vi "Level Function with Limits.vi"() -> ()   [LabVIEW 2014]
panel:
  in  "Bottom":bool
  in  "Top":bool
  out "Motor Value":dbl
  out "Is Below":bool
  out "Is Above":bool
  in  "stop":bool
  out "coerced(x)":dbl
  out "In Range?":bool
  in  "Input":dbl(slide) scale=0.0..20.0
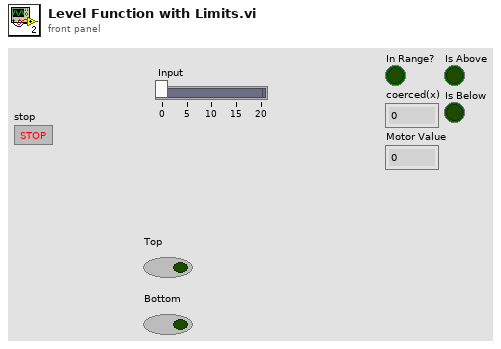
[diagram p1: front panel]
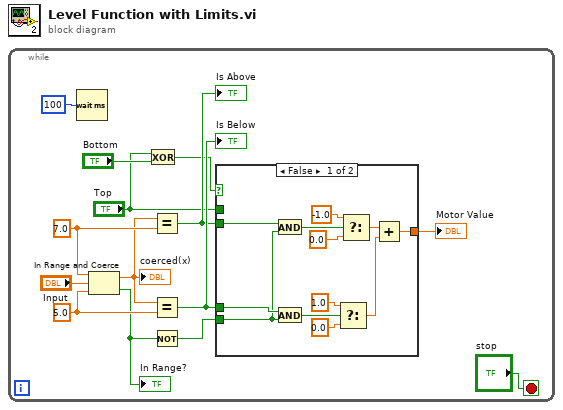
[diagram p0: block diagram]
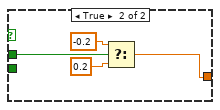
[diagram p2: hidden frame]
diagram:
  n1 = while {
    stop <- "stop" stop-if-true
    w10 = 5.0 ("upper limit")
    w11 = 7.0 ("upper limit")
    n2 = Wait (ms)(milliseconds to wait=u32 100) -> ()  [unwired: 1 out]
    n3 = In Range and Coerce(upper limit=w11, x="Input", lower limit=w10) -> (coerced(x)=w9:dbl, In Range?=w6:bool)
    "In Range?" <- w6
    "coerced(x)" <- w9
    n4 = Exclusive Or(1:"Bottom", 2:"Top") -> (0:w2:bool)
    n5 = Equal?(x=w9, y=w11) -> (x = y?=w7:bool)
    "Is Above" <- w7
    n6 = Equal?(x=w9, y=w10) -> (x = y?=w8:bool)
    "Is Below" <- w8
    n7 = Not(x=w6) -> (.not. x?=w5:bool)
    n8 = case shown="False" w2 {
      tunnel: w8 -> [w17 _]
      tunnel: w7 -> [w18 _]
      tunnel: w5 -> [w16 _]
      tunnel: [w15 w30] -> w4
      tunnel: "Top" -> [_ w29]
      frame False {
        n9 = And(x=w18, y=w16) -> (x .and. y?=w26:bool)
        n10 = And(x=w17, y=w16) -> (x .and. y?=w25:bool)
        n11 = Select(t=1.0, s=w25, f=0.0) -> (s? t:f=w19:dbl)
        n12 = Select(t=-1.0, s=w26, f=0.0) -> (s? t:f=w20:dbl)
        n13 = Add(x=w20, y=w19) -> (x+y=w15:dbl)
      }
      frame True {
        n14 = Select(t=-0.2, s=w29, f=0.2) -> (s? t:f=w30:dbl)
      }
    }
    "Motor Value" <- w4
  }
